vi "分层图显示.vi"(11 "IN":string) -> (3 "OUT":string)   [LabVIEW 2016]
uses:
  <vilib>/Utility/file.llb/Read Delimited Spreadsheet (DBL).vi
panel:
  out "导入完毕？":bool
  in  "ESC":bool
  out "强度图":dbl[][](graph)
  in  "NEXT":bool
  in  "层数:":i32
  out "数组":dbl[][][](array[numeric])
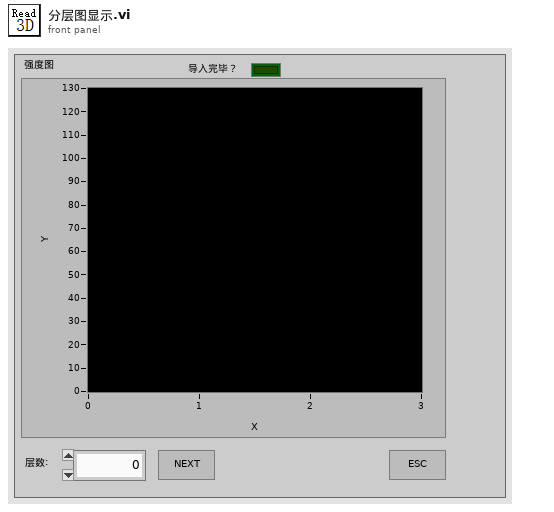
[diagram p1: front panel]
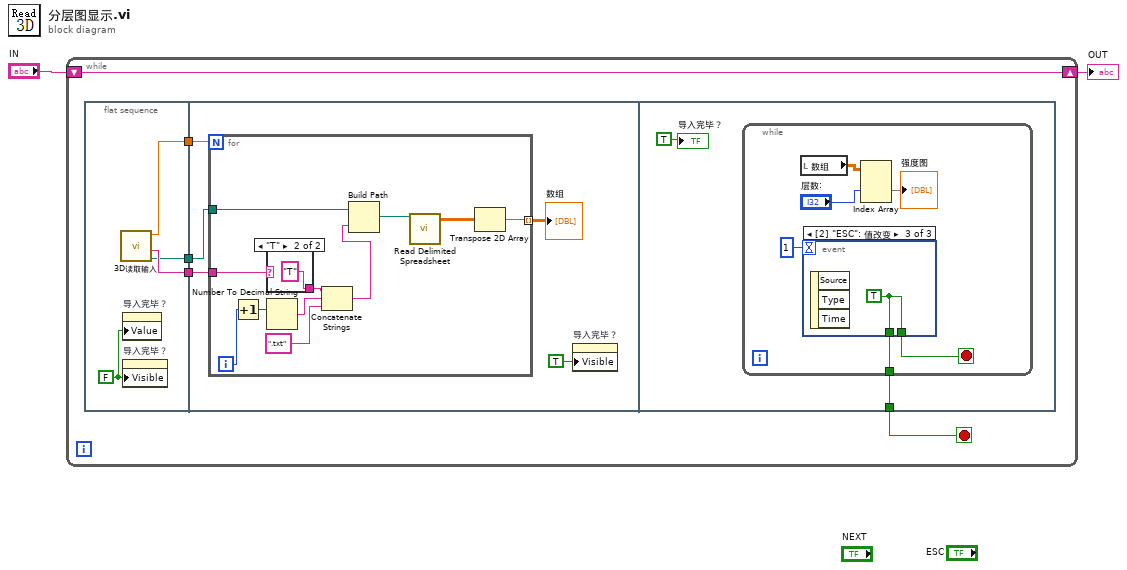
[diagram p0: block diagram]
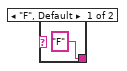
[diagram p2: hidden frame]
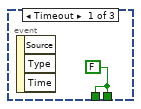
[diagram p3: hidden frame]
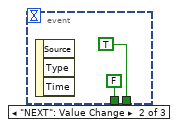
[diagram p4: hidden frame]
diagram:
  n1 = while {
    shift-right: [w4] -> w1
    shift-left: "IN" -> [w4]
    stop <- w3 stop-if-true
    n2 = flat-sequence {
      tunnel: [w11] -> w7
      tunnel: [w10] -> w6
      tunnel: [w9] -> w5
      tunnel: w7 -> [w16]
      tunnel: w6 -> [w15]
      tunnel: w5 -> [w14]
      tunnel: [w31] -> w3
      frame #0 {
        w8 = FALSE ("可见")
        n3 = call "3D读取输入.vi"() -> ("文件读取路径"=w10:path, "时域谱or频域谱"=w11:string, "行总数"=w9:dbl)  [unwired: 9 in]
        n4 = property on="导入完毕？" class="Bool (严格)"("Value"=w8) -> ()  [unwired: 2 in, 2 out]
        n5 = property on="导入完毕？" class="Bool (严格)"("Visible"=w8) -> ()  [unwired: 2 in, 2 out]
      }
      frame #1 {
        n6 = for {
          N: w14 -> [_]
          tunnel: [w26] -> w13 mode=indexing
          tunnel: w16 -> [w18]
          tunnel: w15 -> [w17]
          i -> [w22]
          n7 = Increment(x=w22) -> (x+1=w21:i32)
          n8 = case shown="\"T\"" w18 {
            tunnel: ["F" "T"] -> w24
            frame "F", Default {
            }
            frame "T" {
            }
          }
          n9 = Number To Decimal String(number=w21) -> (decimal integer string=w20:string)  [unwired: 1 in]
          n10 = Concatenate Strings(w24, w20, ".txt") -> (w23:string)
          n11 = Build Path(base path=w17, name or relative path=w23) -> (appended path=w25:path)
          n12 = call-poly <vilib>:"Read Delimited Spreadsheet.vi"("file path (dialog if empty)"=w25) -> ("all rows"=w27:dbl[][])  [unwired: 9 in, 5 out]
          n13 = Transpose 2D Array(2D array=w27) -> (transposed array=w26:dbl[][])
        }
        "数组" <- w13
        n14 = property on="导入完毕？" class="Bool (严格)"("Visible"=TRUE ("可见")) -> ()  [unwired: 2 in, 2 out]
      }
      frame #2 {
        n15 = while {
          tunnel: [w33] -> w31
          stop <- w34 stop-if-true
          n16 = local read "数组"() -> (w37:dbl[][][])
          n17 = event shown="[2] \"ESC\": 值改变" {
            selector: _ -> [_ _ _]
            dyn-events: _ -> [_ _ _]
            timeout: 1 -> [_ _ _]
            tunnel: [w38 TRUE w41] -> w34
            tunnel: [w38 FALSE w41] -> w33
            event Timeout {
              w38 = FALSE
              n18 = event-data() -> ()  [unwired: 1 in, 3 out]
            }
            event "NEXT": Value Change {
              n19 = event-data() -> ()  [unwired: 1 in, 3 out]
            }
            event "ESC": Value Change {
              w41 = TRUE
              n20 = event-data() -> ()  [unwired: 1 in, 3 out]
            }
          }
          n21 = Index Array(array=w37, index (dim 1)="层数:") -> (element=→"强度图":dbl[][])  [unwired: 2 in]
        }
        "导入完毕？" <- TRUE ("导入完毕？")
      }
    }
  }
  "OUT" <- w1
